vi "GPS data to minutes.vi"(1 "GPS Data in (DDmm.mm)":dbl) -> (0 "GPS Data out (in minutes)":dbl)   [LabVIEW 2009]
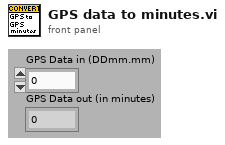
[diagram p1: front panel]
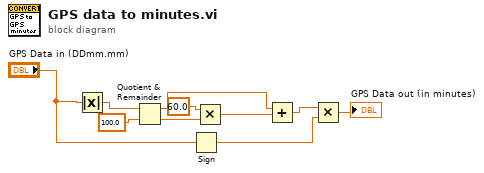
[diagram p0: block diagram]
diagram:
  n1 = Absolute Value(x="GPS Data in (DDmm.mm)") -> (abs(x)=w1:dbl)
  n2 = Quotient & Remainder(x=w1, y=100.0) -> (x-y*floor(x/y)=w7:dbl, floor(x/y)=w9:dbl)
  n3 = Sign(1:"GPS Data in (DDmm.mm)") -> (0:w4:dbl)
  n4 = Multiply(x=60.0, y=w9) -> (x*y=w6:dbl)
  n5 = Add(x=w7, y=w6) -> (x+y=w5:dbl)
  n6 = Multiply(x=w5, y=w4) -> (x*y=→"GPS Data out (in minutes)":dbl)
